vi "Cleanup Read function.vi"(8 "error in (no error)":errorcluster, 9 "Project name":string, 11 "vi reference":refnum<vi>) -> (0 "error out":errorcluster, 3 "vi reference out":refnum<vi>)   [LabVIEW 2018]
doc: "Moves around wires and terminals on the read function to make it prettier."
uses:
  <vilib>/Utility/traverseref.llb/TRef TravTarget.ctl
  <vilib>/Utility/miscctls.llb/LVPointTypeDef.ctl
  <vilib>/Utility/miscctls.llb/LVRectTypeDef.ctl
  <vilib>/Utility/error.llb/Clear Errors.vi
  <userlib>/nLight Error Handling/Log any errors.vi
  <vilib>/Utility/traverseref.llb/VI Scripting - Traverse.lvlib
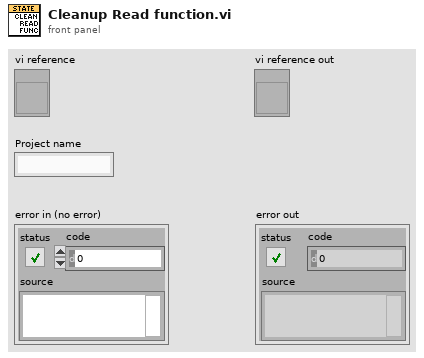
[diagram p1: front panel]
types:
  T1 = typedef "TRef TravTarget.ctl" = enum16{"FP", "BD", "Other"}
  T2 = typedef "LVRectTypeDef.ctl" = cluster{"Left":i16, "Top":i16, "Right":i16, "Bottom":i16}
  T3 = typedef "LVPointTypeDef.ctl" = cluster{"Horizontal":i16, "Vertical":i16}
  T4 = cluster{"Label.Text":string, "Left":i32, "Top":i32}[]
  T5 = cluster{"Label.Text":string, "Left":i32, "Top":i32}
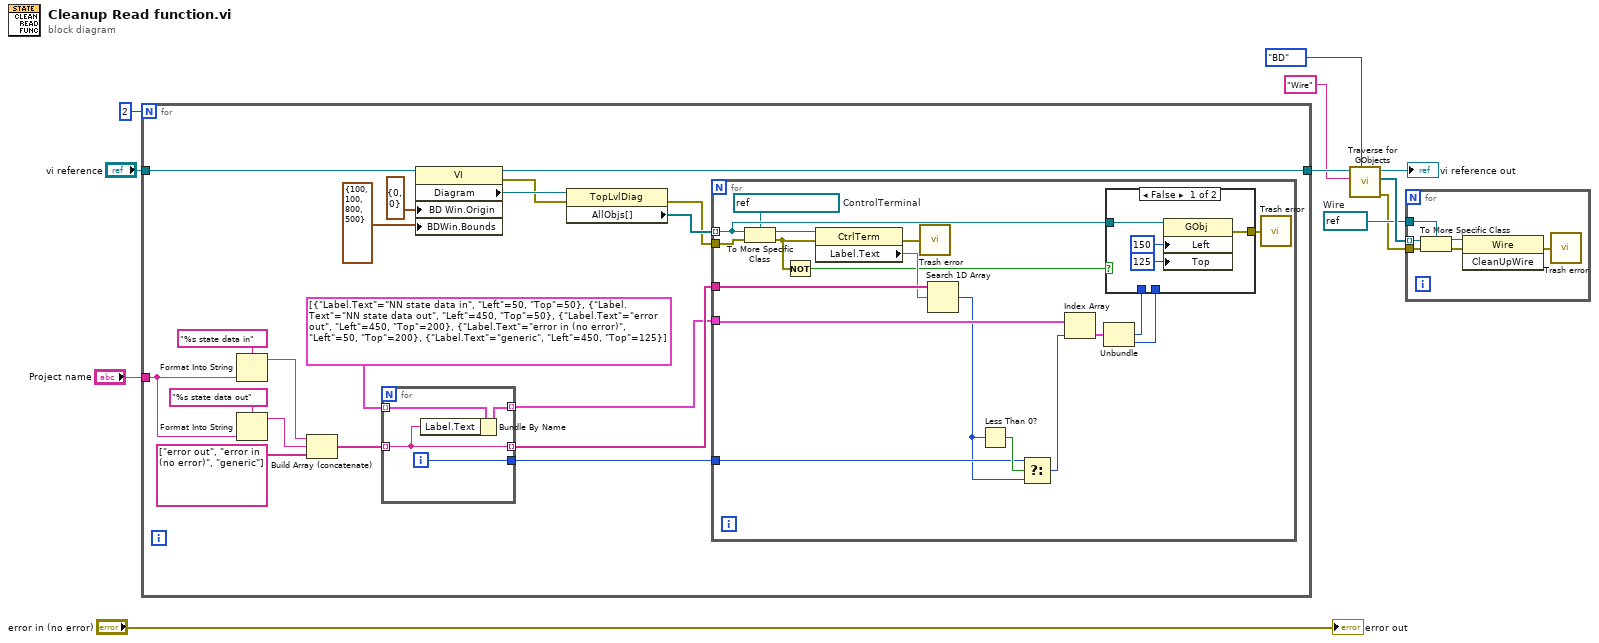
[diagram p0: block diagram]
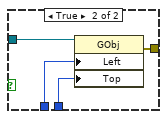
[diagram p2: hidden frame]
diagram:
  w2 = refnum<vi> refnum  # Wire
  n1 = for {
    N: 2 -> [_]
    tunnel: "vi reference" -> [w30]
    tunnel: [w22] -> w9
    tunnel: "Project name" -> [w17]
    n2 = Format Into String(format string="%s state data in" ("Label.Text"), w17) -> (resulting string=w16:string)  [unwired: 2 in, 1 out]
    n3 = Format Into String(format string="%s state data out" ("Label.Text"), w17) -> (resulting string=w15:string)  [unwired: 2 in, 1 out]
    n4 = Build Array (concatenate)(w16, w15, string[] ["error out", "error in (no error)", "generic"] ("Label.Text")) -> (w14:string[])
    n5 = for {
      tunnel: T4 [{"Label.Text"="NN state data in", "Left"=50, "Top"=50}, {"Label.Text"="NN state data out", "Left"=450, "Top"=50}, {"Label.Text"="error out", "Left"=450, "Top"=200}, {"Label.Text"="error in (no error)", "Left"=50, "Top"=200}, {"Label.Text"="generic", "Left"=450, "Top"=125}] ("Array") -> [w34] mode=indexing
      tunnel: [w31] -> w27 mode=indexing
      tunnel: [w32] -> w25
      tunnel: [w33] -> w20 mode=indexing
      tunnel: w14 -> [w31] mode=indexing
      i -> [w32]
      n6 = Bundle By Name(cluster=w34, "Label.Text"=w31) -> (w33:T5)
    }
    n7 = property class="VI"(reference=w30, "BD Win.Origin"=T3 {"Horizontal"=0, "Vertical"=0} ("Block Diagram Window:Origin"), "BDWin.Bounds"=T2 {"Left"=100, "Top"=100, "Right"=800, "Bottom"=500} ("Block Diagram Window:Window Bounds")) -> (reference out=w22:refnum<vi>, error out=w13:errorcluster, "Diagram"=w29:refnum<vi>)  [unwired: 1 in]
    n8 = property class="TopLvlDiag"(reference=w29, error in=w13) -> (error out=w12:errorcluster, "AllObjs[]"=w28:refnum<vi>[])  [unwired: 1 out]
    n9 = for {
      tunnel: w28 -> [w47] mode=indexing
      tunnel: w20 -> [w49]
      tunnel: w27 -> [w51]
      tunnel: w25 -> [w42]
      tunnel: w12 -> [w38]
      w39 = refnum<vi> refnum  # ControlTerminal
      n10 = To More Specific Class(target class=w39, reference=w47, error in=w38) -> (specific class reference=w52:refnum<vi>, error out=w37:errorcluster)
      n11 = Not(x=w37) -> (.not. x?=w44:bool)
      n12 = property class="CtrlTerm"(reference=w52, error in=w37) -> (error out=w36:errorcluster, "Label.Text"=w50:string)  [unwired: 1 out]
      n13 = call <userlib>:"Trash error.vi"("error in"=w36) -> ()  [unwired: 15 in]
      n14 = Search 1D Array(1D array=w51, element=w50) -> (index of element=w41:i32)  [unwired: 1 in]
      n15 = Less Than 0?(x=w41) -> (x < 0?=w43:bool)
      n16 = Select(t=w42, s=w43, f=w41) -> (s? t:f=w40:i32)
      n17 = Index Array(array=w49, index=w40) -> (element=w48:T5)
      n18 = Unbundle(w48) -> ("Left"=w46:i32, "Top"=w45:i32)  [unwired: 1 out]
      n19 = case shown="False" w44 {
        tunnel: w47 -> [w56 w60]
        tunnel: w46 -> [_ w59]
        tunnel: w45 -> [_ w58]
        tunnel: [w53 w57] -> w35
        frame False {
          n20 = property class="GObj"(reference=w56, "Left"=150 ("Position:Left"), "Top"=125 ("Position:Top")) -> (error out=w53:errorcluster)  [unwired: 1 in, 1 out]
        }
        frame True {
          n21 = property class="GObj"(reference=w60, "Left"=w59, "Top"=w58) -> (error out=w57:errorcluster)  [unwired: 1 in, 1 out]
        }
      }
      n22 = call <userlib>:"Trash error.vi"("error in"=w35) -> ()  [unwired: 15 in]
    }
  }
  n23 = call <vilib>:"Traverse for GObjects.vi"("Traverse Target"=TRef_TravTarget."BD", "Class Name"="Wire", "VI Refnum"=w9) -> ("error out"=w1:errorcluster, "References"=w3:refnum<vi>[], "dup VI Refnum"=→"vi reference out":refnum<vi>)  [unwired: 5 in, 1 out]
  n24 = for {
    tunnel: w3 -> [w66] mode=indexing
    tunnel: w2 -> [w65]
    tunnel: w1 -> [w61]
    n25 = To More Specific Class(target class=w65, reference=w66, error in=w61) -> (specific class reference=w63:refnum<vi>, error out=w64:errorcluster)
    n26 = invoke class="Wire" method="CleanUpWire"(reference=w63, error in=w64) -> (error out=w62:errorcluster)  [unwired: 1 in, 2 out]
    n27 = call <userlib>:"Trash error.vi"("error in"=w62) -> ()  [unwired: 15 in]
  }
  "error out" <- "error in (no error)"
